vi "read_trial_sequence.vi"(8 "error in (no error)":errorcluster, 11 "file path":path) -> (0 "error out":errorcluster, 3 "Array":i32[][][](array[numeric]))   [LabVIEW 2012]
uses:
  utilities/labview/read_matrix_reshape_3D.vi
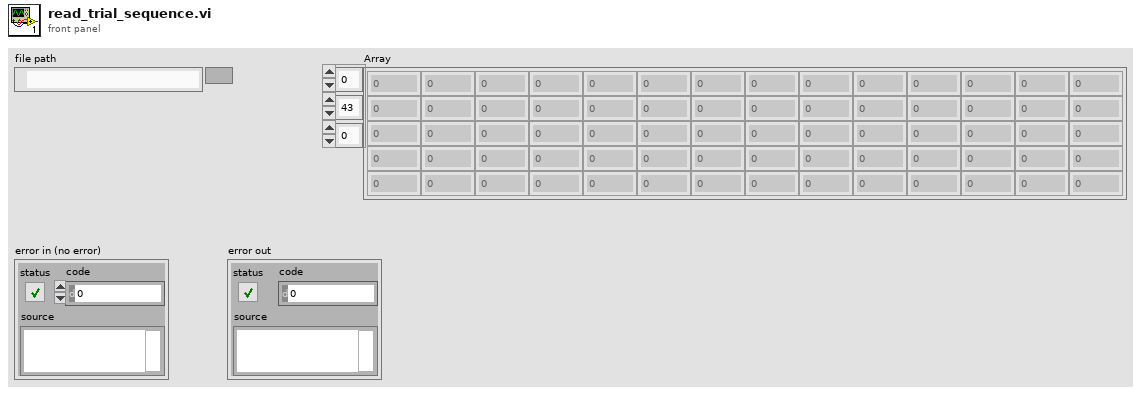
[diagram p1: front panel]
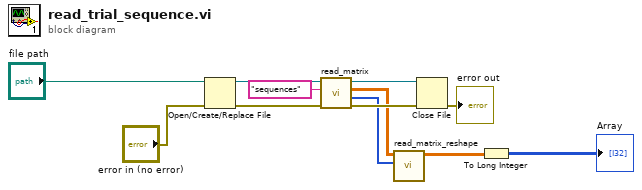
[diagram p0: block diagram]
diagram:
  n1 = Open/Create/Replace File(file path (use dialog)="file path", error in="error in (no error)") -> (refnum out=w3:refnum<file>, error out=w5:errorcluster)  [unwired: 4 in, 1 out]
  n2 = call "read_matrix.vi"("error in"=w5, "Entry name"="sequences", "file refnum"=w3) -> ("error out"=w10:errorcluster, "Dimensions"=w8:i32[], "Result"=w7:dbl[][], "refnum out"=w9:refnum<file>)  [unwired: 4 in, 1 out]
  n3 = call-poly "read_matrix_reshape.vi"("Dimensions"=w8, "Result in"=w7) -> ("Result out"=w12:dbl[][][])  [unwired: 9 in]
  n4 = Close File(refnum=w9, error in=w10) -> (error out=→"error out":errorcluster)  [unwired: 1 out]
  n5 = To Long Integer(number=w12) -> (32bit integer=→"Array":i32[][][])
